vi "LakeShore Conditional Save.vi"(0 "VISA session":refnum<visa-resource-name>, 1 "340? and changed":bool) -> (2 "dup VISA session":refnum<visa-resource-name>)   [LabVIEW 2024]
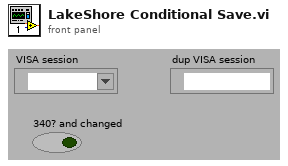
[diagram p1: front panel]
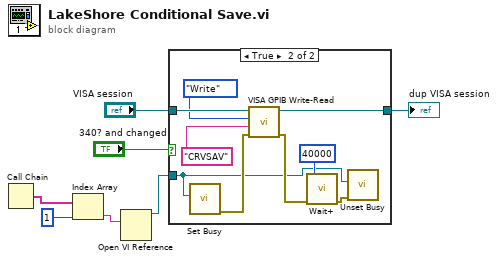
[diagram p0: block diagram]
diagram:
  n1 = Call Chain() -> (call chain=w4:string[])
  n2 = Index Array(array=w4, index=1) -> (element=w2:string)
  n3 = Open VI Reference(vi path=w2) -> (vi reference=w1:refnum<vi>)  [unwired: 5 in, 1 out]
  n4 = case shown="True" "340? and changed" {
    tunnel: "VISA session" -> [w8 w17]
    tunnel: [w8 w16] -> w7
    tunnel: w1 -> [_ w9]
    frame False {
    }
    frame True {
      n5 = call <vilib>:"Set Busy.vi"("VI reference (current VI)"=w9) -> ("error out"=w13:errorcluster)  [unwired: 9 in, 1 out]
      n6 = call "VISA GPIB Write-Read.vi"("error in (no error)"=w13, "Command"="CRVSAV" ("String to Write"), "Action"=enum16{"Write", "Read", "Write & Read"}."Write", "VISA resource name"=w17) -> ("error out"=w12:errorcluster, "dup VISA Session"=w16:refnum<visa-resource-name>)  [unwired: 4 in, 2 out]
      n7 = call "Wait+.vi"("Error In"=w12, "milliseconds to wait"=u32 40000) -> ("Error Out"=w11:errorcluster)  [unwired: 4 in, 1 out]
      n8 = call <vilib>:"Unset Busy.vi"("error in (no error)"=w11, "VI reference (current VI)"=w9) -> ()  [unwired: 9 in, 1 out]
    }
  }
  "dup VISA session" <- w7
